vi "cam_dll_test2.vi"() -> ()   [LabVIEW 2013]
panel:
  out "써머커플":dbl=41.98981437935929
  out "최대값":dbl=42.12532958984377
  out "슬라이드":i32(slide)=153 scale=0.0..320.0
  out "강도 그래프":dbl[][](graph)
  in  "y":i32=256
  in  "x":i32=320
  in  "STOP":bool=TRUE
  in  "IPadderss":string="169.254.96.112"
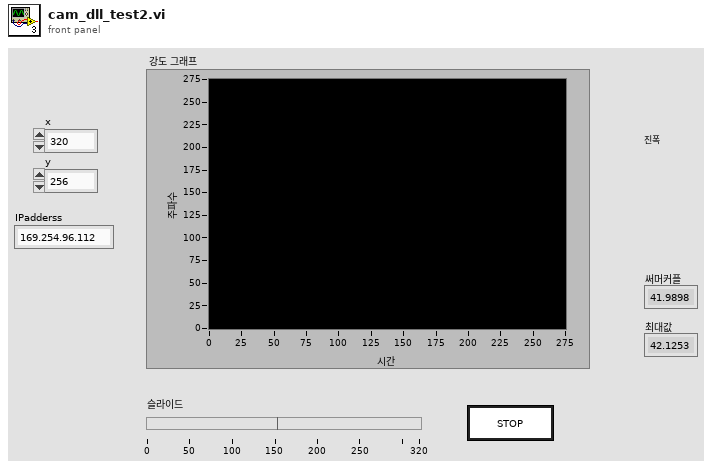
[diagram p1: front panel]
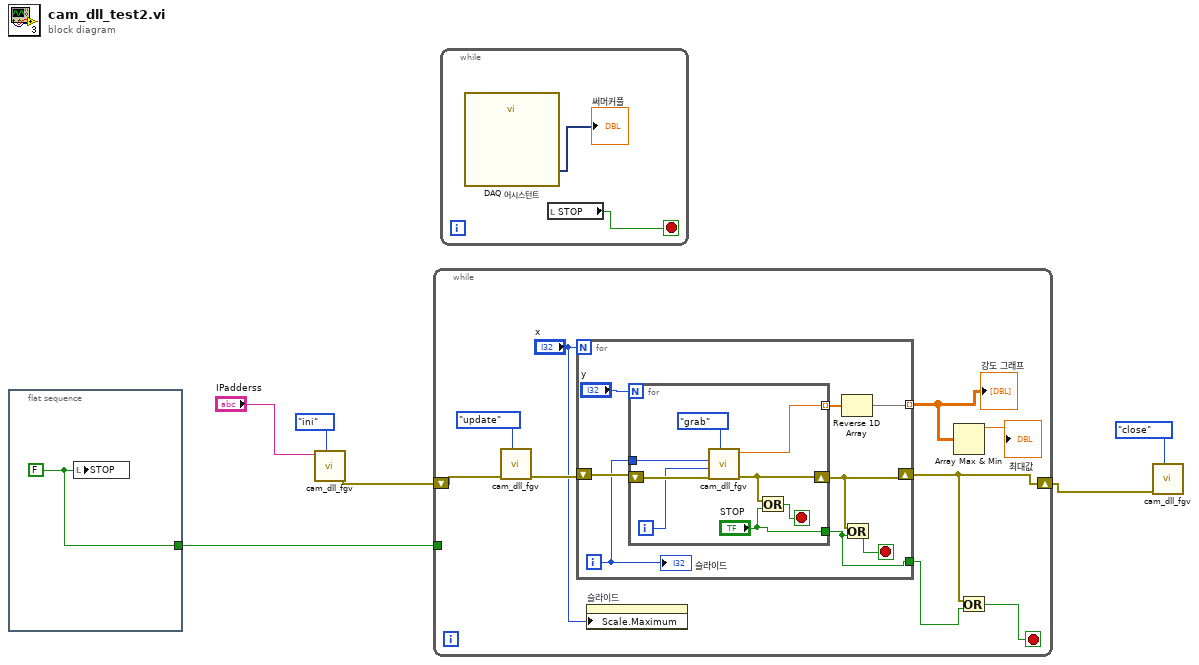
[diagram p0: block diagram]
diagram:
  n1 = flat-sequence {
    tunnel: [w7] -> w1
    frame #0 {
      w7 = FALSE ("STOP")
      n2 = local write "STOP"(w7) -> ()
    }
  }
  n3 = call "cam_dll_fgv.vi"("cmd"=enum16{"update", "grab", "ini", "close"}."ini", "IPadderss"="IPadderss") -> ("error out"=w4:errorcluster)  [unwired: 8 in, 1 out]
  n4 = while {
    shift-right: [w12] -> w2
    shift-left: w4 -> [w15]
    tunnel: w1 -> [_]
    stop <- w13 stop-if-true
    n5 = call "cam_dll_fgv.vi"("cmd"=enum16{"update", "grab", "ini", "close"}."update", "error in"=w15) -> ("error out"=w14:errorcluster)  [unwired: 8 in, 1 out]
    n6 = for {
      N: "x" -> [_]
      shift-right: [w19] -> w12
      shift-left: w14 -> [w24]
      tunnel: [w21] -> w10 mode=indexing
      tunnel: [w17] -> w8
      i -> [w20]
      stop <- w18 stop-if-true
      n7 = for {
        N: "y" -> [_]
        shift-right: [w27] -> w19
        shift-left: w24 -> [w31]
        tunnel: w20 -> [w29]
        tunnel: [w30] -> w22 mode=indexing
        tunnel: ["STOP"] -> w17
        i -> [w28]
        stop <- w26 stop-if-true
        n8 = call "cam_dll_fgv.vi"("cmd"=enum16{"update", "grab", "ini", "close"}."grab", "error in"=w31, "nYposition"=w28, "nXposition"=w29) -> ("error out"=w27:errorcluster, "temp"=w30:dbl)  [unwired: 6 in]
        n9 = Or(x=w27, y="STOP") -> (x .or. y?=w26:bool)
      }
      n10 = Reverse 1D Array(array=w22) -> (reversed array=w21:dbl[])
      n11 = Or(x=w19, y=w17) -> (x .or. y?=w18:bool)
      "슬라이드" <- w20
    }
    "강도 그래프" <- w10
    n12 = property on="슬라이드" class="Slide (엄격한)"("Scale.Maximum"="x") -> ()  [unwired: 2 in, 2 out]
    n13 = Array Max & Min(array=w10) -> (max value=→"최대값":dbl)  [unwired: 3 out]
    n14 = Or(x=w12, y=w8) -> (x .or. y?=w13:bool)
  }
  n15 = while {
    stop <- w34 stop-if-true
    n16 = call "DAQ 어시스턴트"() -> ("data"=→"써머커플":dynamicdata)  [unwired: 17 in, 2 out]
    n17 = local read "STOP"() -> (w34:bool)
  }
  n18 = call "cam_dll_fgv.vi"("cmd"=enum16{"update", "grab", "ini", "close"}."close", "error in"=w2) -> ()  [unwired: 8 in, 2 out]
